vi "Handle Error.vi"(8 "error in (no error)":errorcluster, 11 "Abstract Sensor Interface in":refnum<class "Abstract Sensor Interface.lvclass">) -> (0 "error out":errorcluster, 2 "stop actor?":bool=TRUE, 3 "Abstract Sensor Interface out":refnum<class "Abstract Sensor Interface.lvclass">)   [LabVIEW 2019, in "Abstract Sensor Interface Actor.lvlib" / "Abstract Sensor Interface.lvclass"]
doc: "(<B>Filename</B>: Actor Framework.lvlib:Actor.lvclass:Handle Error.vi)\n\nDefines how the actor handles an error that occurred while processing a message. By default, this method does nothing except stop the actor."
uses:
  Abstract Sensor Interface.lvclass
  <vilib>/ActorFramework/Actor/Actor.lvclass
  Elevator Controller Actor/Elevator Controller Messages/Centrize Error Handler Msg/Centrize Error Handler Msg.lvclass
  Elevator Controller Actor/Elevator Controller Messages/Set State Msg/Set State Msg.lvclass
  Elevator Controller Actor/Elevator Control Actor/States -Enum.ctl
  Elevator Controller Actor/Elevator Control Actor/Elevator Controller.lvclass
  C:/Program Files (x86)/National Instruments/LabVIEW 2019/vi.lib/ActorFramework/Actor/Actor.lvclass
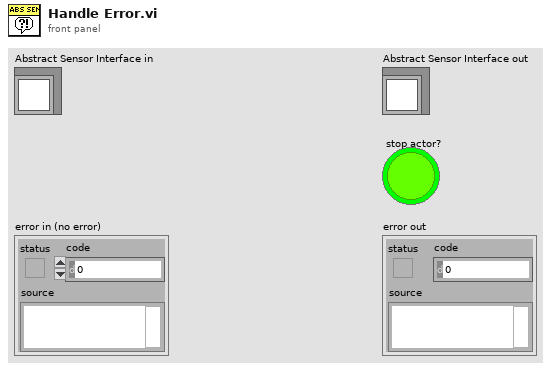
[diagram p1: front panel]
types:
  T1 = typedef "Elevator Controller Actor.lvlib/Elevator Controller.lvclass/States -Enum.ctl" = enum16{"Initial State", "Start and Move State", "Analysis State", "Continue Travel State", "Open and Close Door Sequence", "Stop at Floor", "No Request remaining", "Emergency Call", "Terminate Process"}
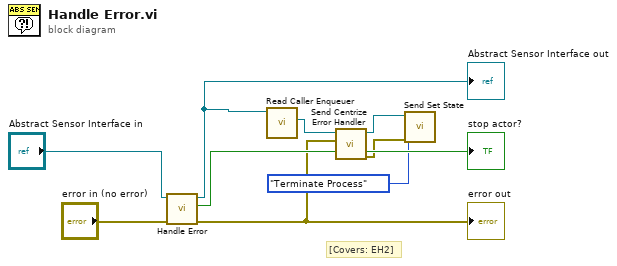
[diagram p0: block diagram]
diagram:
  # "[Covers: EH2]"
  n1 = call-parent "Handle Error.vi"("error in (no error)"="error in (no error)", "Actor in"="Abstract Sensor Interface in") -> ("error out"=w4:errorcluster, "stop actor?"=→"stop actor?":bool, "Actor out"=w5:refnum<class "Abstract Sensor Interface.lvclass">)  [unwired: 7 in]
  "Abstract Sensor Interface out" <- w5
  "error out" <- w4
  n2 = call <vilib>:"Read Caller Enqueuer.vi"("Actor"=w5) -> ("Caller Enqueuer"=w6:refnum<class "Message Enqueuer.lvclass">)  [unwired: 10 in]
  n3 = call "Send Centrize Error Handler.vi"("Error"=w4, "Message Enqueuer"=w6) -> ("error out"=w1:errorcluster, "Message Enqueuer out"=w3:refnum<class "Message Enqueuer.lvclass">)  [unwired: 8 in]
  n4 = call "Send Set State.vi"("error in (no error)"=w1, "States"=States_-Enum."Terminate Process", "Message Enqueuer"=w3) -> ()  [unwired: 7 in, 2 out]
